vi "InverseMagnetics.vi"(6 "Bz [T]":dbl, 7 "X (m)":dbl, 8 "By [T]":dbl, 9 "Bx [T]":dbl, 10 "Z (m)":dbl, 11 "Y (m)":dbl) -> (0 "ZN":dbl, 1 "YP":dbl, 2 "YN":dbl, 3 "XP":dbl, 4 "ZP":dbl, 5 "XN":dbl)   [LabVIEW 2017]
uses:
  Documents/LabVIEW Data/MathScriptVIs/MCStatic_38590875332_2924ca3c37852a9d2934950055dc824a.vi
  <instcachedir>/0/MCStatic_38590875332_2924ca3c37852a9d2934950055dc824a_CAEBCB76FA154702AEF5C1A9DA0D3E2B.lvgen/MCStatic_38590875332_2924ca3c37852a9d2934950055dc824a_CAEBCB76FA154702AEF5C1A9DA0D3E2B_000.vi
  <vilib>/imath/engines/lvmath2/RunTimeEngine/IndexRead/NIMS V(S).vi
  <instcachedir>/0/NIMS V(S)_0488751826AF41519A22953C041130DC.lvgen/NIMS V(S)_0488751826AF41519A22953C041130DC_003.vi
  <vilib>/imath/engines/lvmath2/RunTimeEngine/ErrorHandling/NIMS_Create Error From Enums.vi
  <vilib>/imath/engines/lvmath2/RunTimeEngine/ArithmeticOperatorToken/NIMS_ArithmeticOperator_multmx-internal.vi
  <instcachedir>/0/NIMS_ArithmeticOperator_multmx-internal_D14B0E8358F948B18FBB33DB0D4CACE1.lvgen/NIMS_ArithmeticOperator_multmx-internal_D14B0E8358F948B18FBB33DB0D4CACE1_003.vi
  <vilib>/imath/engines/lvmath2/RunTimeEngine/ArithmeticOperatorToken/NIMS_ArithmeticOperator_rightdivmx(C,C)-internal.vi
  <instcachedir>/0/NIMS_ArithmeticOperator_rightdivmx(C,C)-internal_F4E363C546B1452B989A7C6F3BFC253B.lvgen/NIMS_ArithmeticOperator_rightdivmx(C,C)-internal_F4E363C546B1452B989A7C6F3BFC253B_000.vi
  <vilib>/imath/engines/lvmath2/RunTimeEngine/ArithmeticOperatorToken/NIMS_ArithmeticOperator_multmx(M,CV)-internal.vi
  <instcachedir>/0/NIMS_ArithmeticOperator_multmx(M,CV)-internal_5132FFBA5DFA43CC8541399EB82087B3.lvgen/NIMS_ArithmeticOperator_multmx(M,CV)-internal_5132FFBA5DFA43CC8541399EB82087B3_003.vi
  <vilib>/imathl/engines/lvmath/Functions/Error Handling/Create Error.vi
  <vilib>/imath/engines/lvmath2/RunTimeEngine/NodeEndStatement/NIMS_NodeEndStatement_Output.vi
  <instcachedir>/0/NIMS_NodeEndStatement_Output_53EC0D466D134D7ABD903AC30B43404B.lvgen/NIMS_NodeEndStatement_Output_53EC0D466D134D7ABD903AC30B43404B_009.vi
  <vilib>/imath/engines/lvmath2/RunTimeEngine/ErrorHandling/NIMS_Finalize Error.vi
  MatlabFunctions/GFunction.m
panel:
  # "Current in each coil (A)"
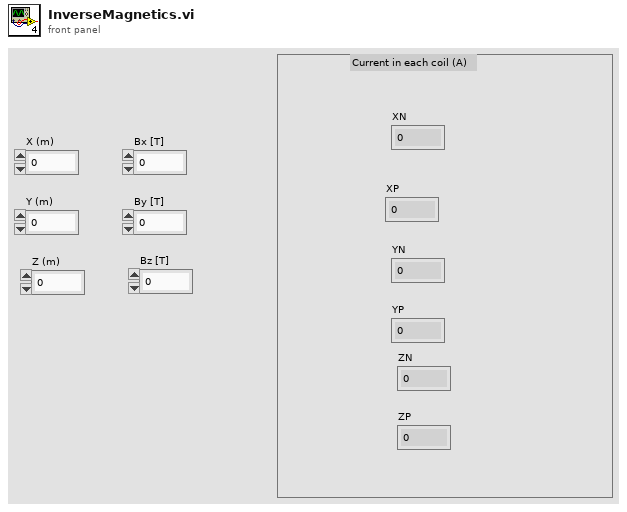
[diagram p1: front panel]
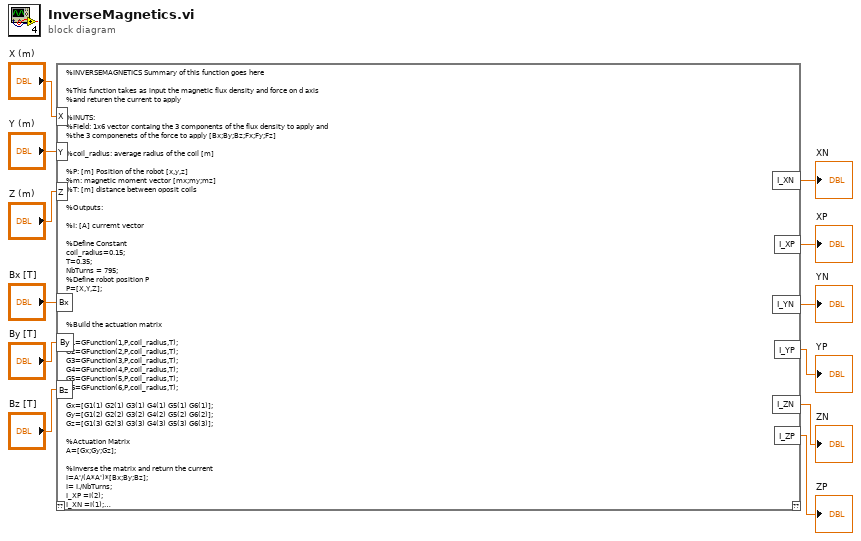
[diagram p0: block diagram]
diagram:
  n1 = mathscript code="%INVERSEMAGNETICS Summary of this function goes here\n\n%This function takes as input the magnetic flux density and force on d axis\n%and returen the current to apply\n\n%INUTS: \n%Field: 1x6 vector containg the 3 components of the flux density to apply and\n%the 3 componenets of the force to apply [Bx;By;Bz;Fx;Fy;Fz]\n\n%coil_radius: average radius of the coil [m]\n\n%P: [m] Position of the robot [x,y,z]\n%m: magnetic moment vector [mx;my;mz]\n%T: [m] distance between oposit coils\n\n%Outputs: \n\n%I: [A] curremt vector\n\n%Define Constant\ncoil_radius=0.15;\nT=0.35;\nNbTurns = 795;\n%Define robot position P\nP=[X,Y,Z];\n\n\n\n%Build the actuation matrix \n\nG1=GFunction(1,P,coil_radius,T);\nG2=GFunction(2,P,coil_radius,T);\nG3=GFunction(3,P,coil_radius,T);\nG4=GFunction(4,P,coil_radius,T);\nG5=GFunction(5,P,coil_radius,T);\nG6=GFunction(6,P,coil_radius,T);\n\nGx=[G1(1) G2(1) G3(1) G4(1) G5(1) G6(1)];\nGy=[G1(2) G2(2) G3(2) G4(2) G5(2) G6(2)];\nGz=[G1(3) G2(3) G3(3) G4(3) G5(3) G6(3)];\n\n%Actuation Matrix\nA=[Gx;Gy;Gz];\n\n%Inverse the matrix and return the current\nI=A'/(A*A')*[Bx;By;Bz];\nI= I./NbTurns;\nI_XP =I(2);\nI_XN =I(1);\nI_YP =I(4);\nI_YN =I(3);\nI_ZP =-I(6);\nI_ZN =I(5);"("X"="X (m)", "Y"="Y (m)", "Z"="Z (m)", "Bx"="Bx [T]", "By"="By [T]", "Bz"="Bz [T]") -> ("I_XN"=→"XN":cdb, "I_XP"=→"XP":cdb, "I_YN"=→"YN":cdb, "I_YP"=→"YP":cdb, "I_ZN"=→"ZN":cdb, "I_ZP"=→"ZP":cdb)  [unwired: 1 in, 1 out]
